vi "Frame.Dialog.vi"(6 "Signals":T1[](array[typedef]) {"Byte Order" items=["Little Endian", "Big Endian"]; "Data Type" items=["Signed", "Unsigned", "IEEE Float"]}, 7 "Show Name&ID":bool=TRUE, 8 "error in (no error)":errorcluster, 9 "ID":u16=1 caption="ID/Address" min=1 format="%.0x", 10 "Existing PIDs":string[](array[string]), 11 "Name":string) -> (0 "error out":errorcluster, 1 "ID out":u16=1 min=1 format="%.0x", 2 "Cancel PID?":bool, 3 "Name out":string, 4 "Signals out":T1[](array[typedef]) {"Byte Order" items=["Little Endian", "Big Endian"]; "Data Type" items=["Signed", "Unsigned", "IEEE Float"]})   [LabVIEW 2015, in "Diagnostics Addon System Explorer.lvlib"]
uses:
  Diagnostics Addon System Explorer.lvlib
  Shared/Types/Signal.ctl
  <vilib>/NI/AMC/Create Single Message.vi
  <vilib>/NI/AMC/Update Message Routing Info.vi
  <vilib>/NI/AMC/Read Termination Message.vi
  <vilib>/NI/AMC/Send Message.vi
  <vilib>/NI/AMC/Globals.vi
  Shared/Diagnostics Addon Shared.lvlib
  <vilib>/NI/AMC/AMC.lvlib
panel:
  in  "Default":dbl format="%g"
  in  "Units":string
  in  "Endian":u8(ring) items=["Little", "Big"]
  in  "Datatype":u8(ring)=1 items=["Signed", "Unsigned", "Float"]
  in  "Remove":bool
  in  "Add":bool
  in  "Cancel PID":bool
  in  "Apply":bool
  in  "Cancel":bool
  in  "OK":bool
  in  "Maximum":dbl=255.0 format="%g"
  in  "Minimum":dbl format="%g"
  in  "Offset":dbl format="%g"
  in  "Factor":dbl=1.0 format="%g"
  in  "Length":u32=8
  in  "Start Bit":u32
  in  "Signal Name":string
  in  "Signals":i32(listbox)
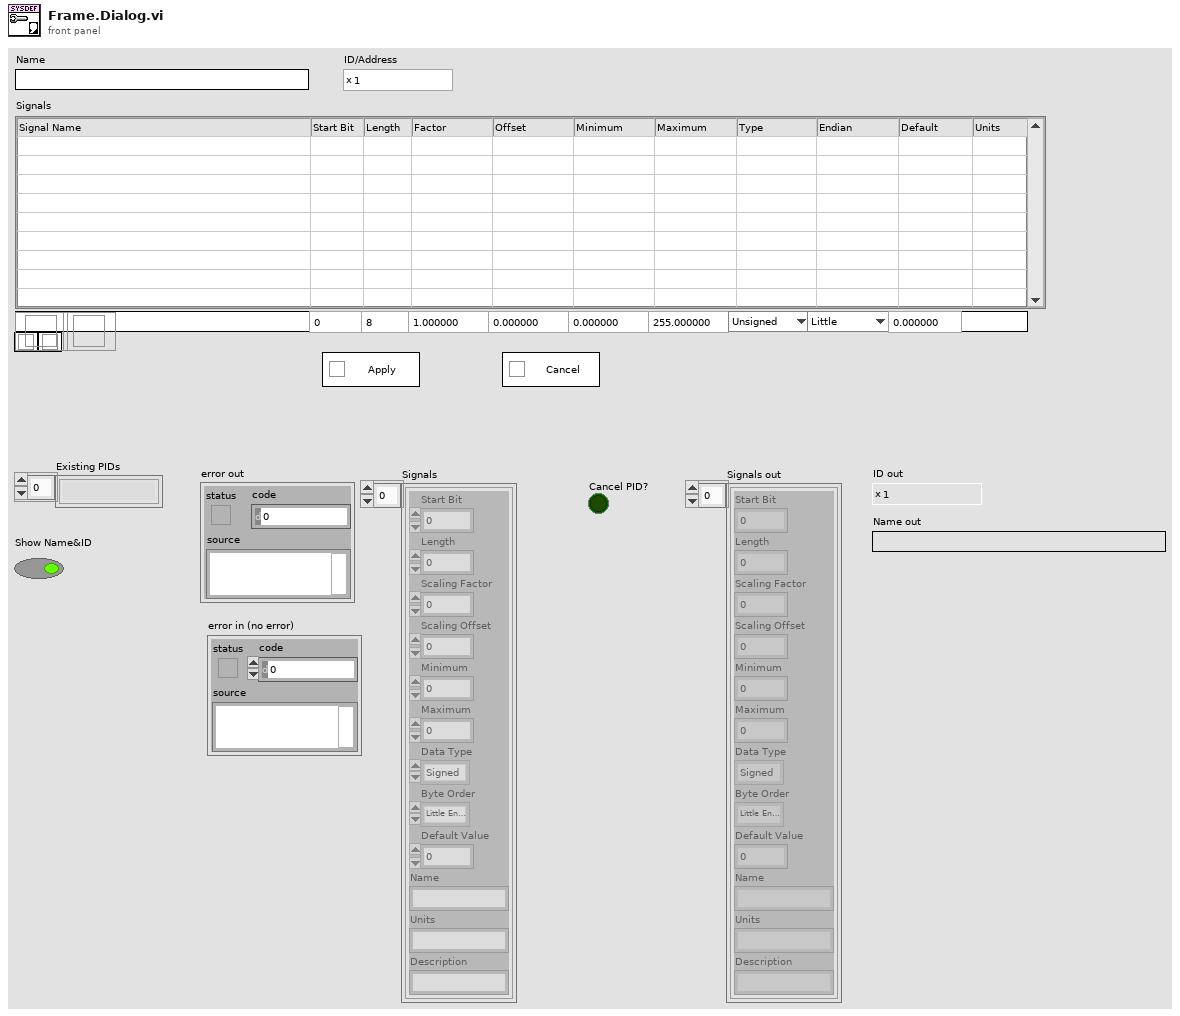
[diagram p1: front panel]
types:
  T1 = typedef "Diagnostics Addon Shared.lvlib/Signal.ctl" = cluster{"Start Bit":u32, "Length":u32, "Scaling Factor":dbl, "Scaling Offset":dbl, "Minimum":dbl, "Maximum":dbl, "Data Type":u32, "Byte Order":u32, "Default Value":dbl, "Name":string, "Units":string, "Description":string}
  T2 = cluster{"NewControlRefs":refnum<vi>[], "Add":refnum<vi>, "Listbox":refnum<vi>, "Remove":refnum<vi>, "Apply":refnum<vi>, "Cancel PID":refnum<vi>}
  T3 = typedef "AMC.lvlib/Message Queue.ctl" = refnum<queue>
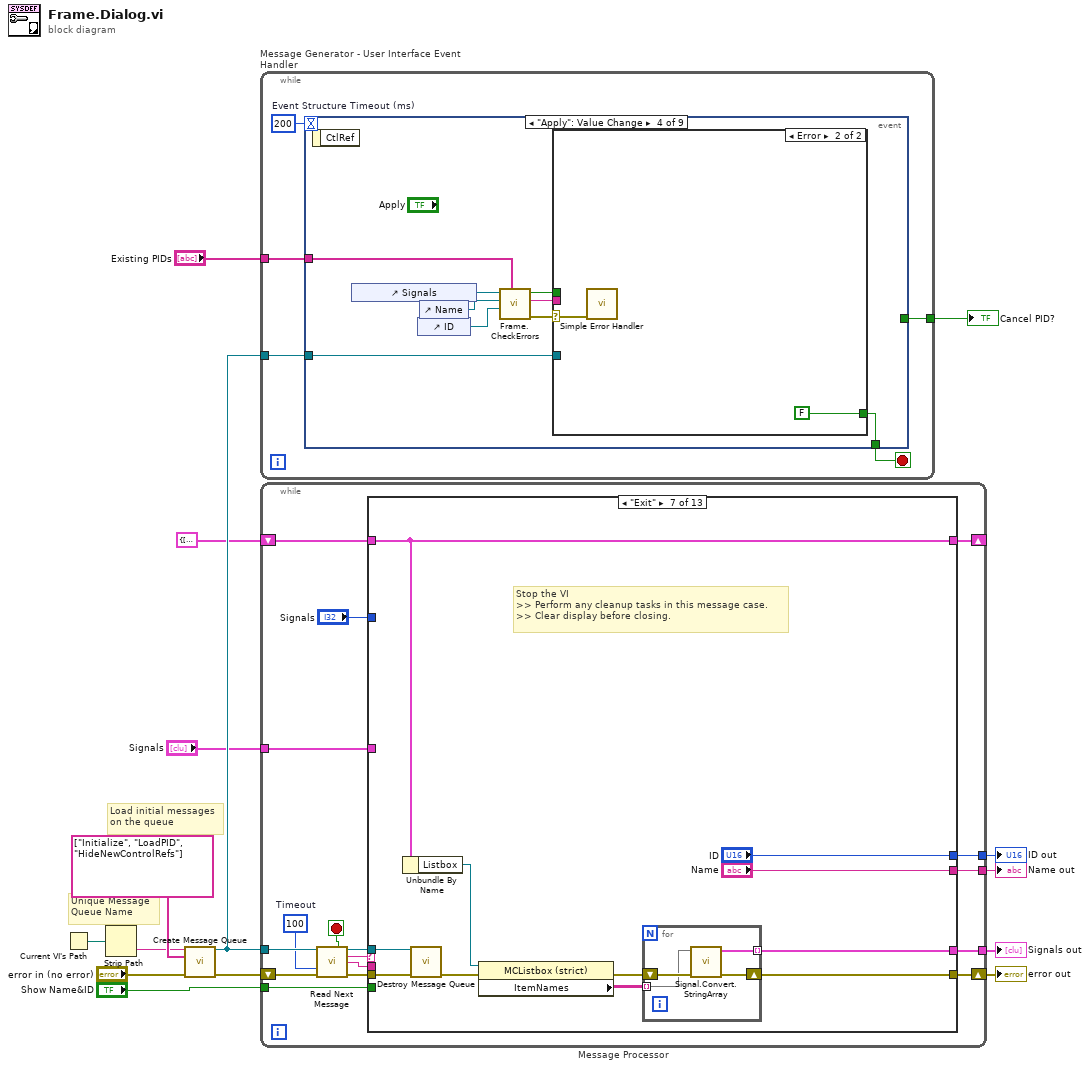
[diagram p0: block diagram]
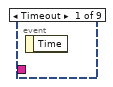
[diagram p2: hidden frame]
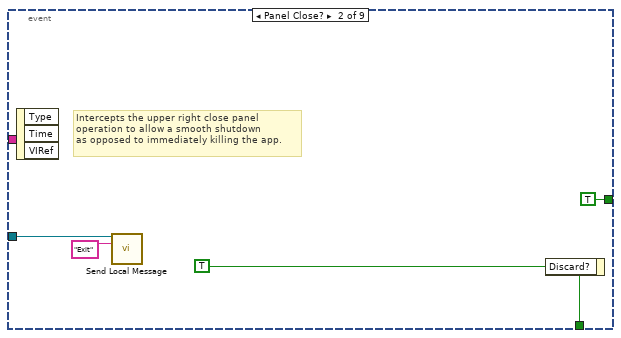
[diagram p3: hidden frame]
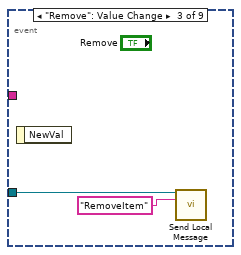
[diagram p4: hidden frame]
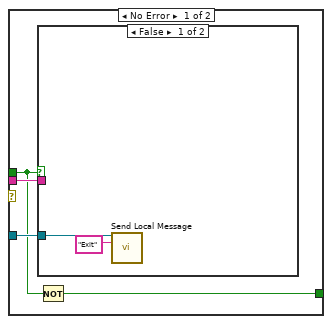
[diagram p5: hidden frame]
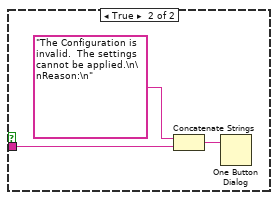
[diagram p6: hidden frame]
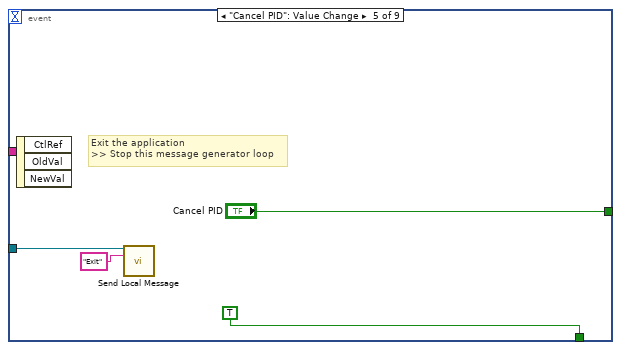
[diagram p7: hidden frame]
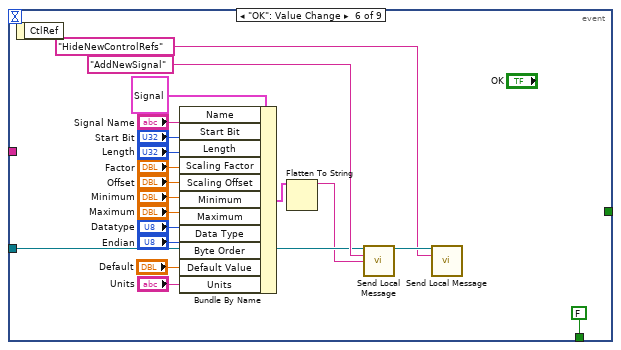
[diagram p8: hidden frame]
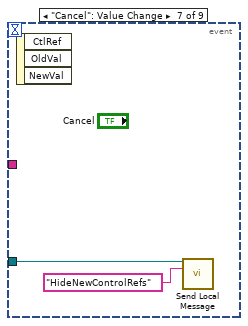
[diagram p9: hidden frame]
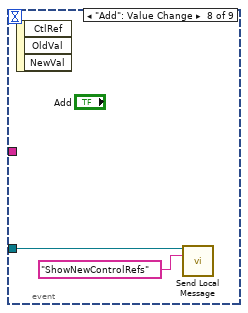
[diagram p10: hidden frame]
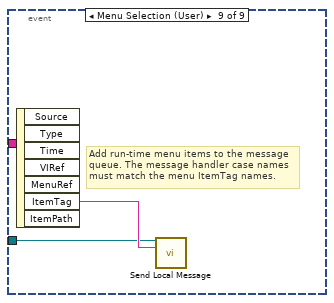
[diagram p11: hidden frame]
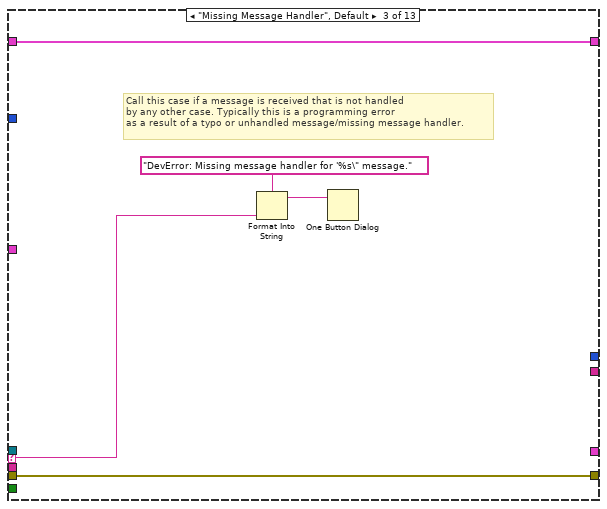
[diagram p14: hidden frame]
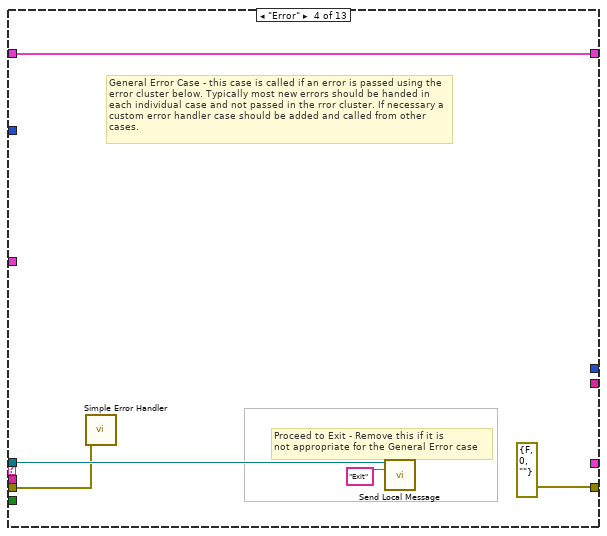
[diagram p15: hidden frame]
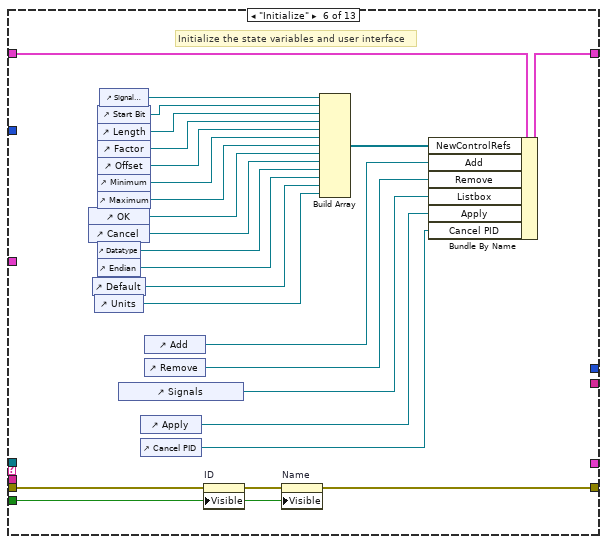
[diagram p17: hidden frame]
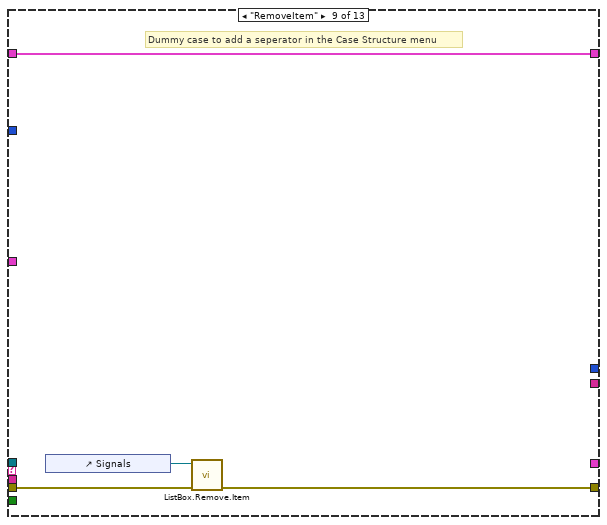
[diagram p19: hidden frame]
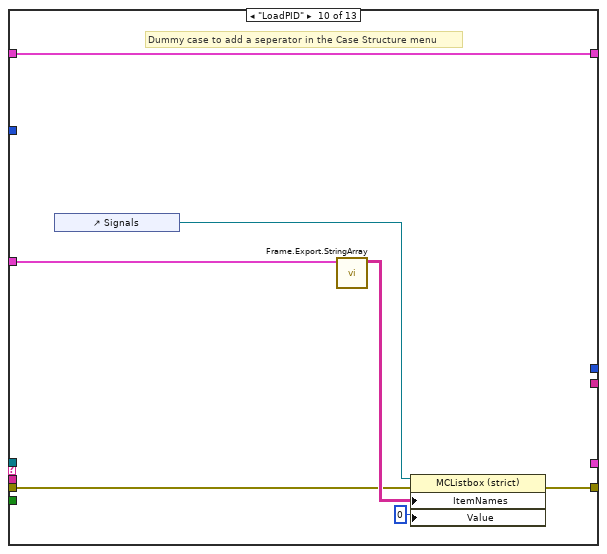
[diagram p20: hidden frame]
diagram:
  # "Unique Message\nQueue Name"
  # "Load initial messages\non the queue"
  n1 = Current VI's Path() -> (path=w11:path)
  n2 = Strip Path(path=w11) -> (name=w14:string)  [unwired: 1 out]
  n3 = call <vilib>:"Create Message Queue.vi"("message queue name"=w14, "initial message names"=string[] ["Initialize", "LoadPID", "HideNewControlRefs"], "error in"="error in (no error)") -> ("message queue out"=w13:T3, "error out"=w12:errorcluster)  [unwired: 11 in]
  n4 = while "Message Generator - User Interface Event Handler" {
    tunnel: w13 -> [w18]
    tunnel: [w17] -> w9
    tunnel: "Existing PIDs" -> [w16]
    stop <- w19 stop-if-true
    w20 = 200  # Event Structure Timeout (ms)
    n5 = event shown="[3] \"Apply\": Value Change" {
      selector: _ -> [_ _ _ _ _ _ _ _ _]
      dyn-events: _ -> [_ _ _ _ _ _ _ _ _]
      timeout: w20 -> [_ _ _ _ _ _ _ _ _]
      tunnel: [_ w24 _ w27 TRUE ("Discard?") FALSE ("Discard?") _ _ _] -> w19
      tunnel: w18 -> [_ w22 w25 w33 w48 w67 w70 w72 w74]
      tunnel: [_ TRUE ("Cancel PID") _ _ "Cancel PID" _ _ _ _] -> w17
      tunnel: w16 -> [_ _ _ w30 _ _ _ _ _]
      event Timeout {
        n6 = event-data() -> ()  [unwired: 2 out]
      }
      event Panel Close? {
        w24 = TRUE ("Discard?")
        # "Intercepts the upper right close panel\noperation to allow a smooth shutdown\nas opposed to immediately killing the app."
        n7 = event-data() -> ()  [unwired: 4 out]
        n8 = call <vilib>:"Send Local Message.vi"("message queue in"=w22, "message name"="Exit") -> ()  [unwired: 11 in, 3 out]
        n9 = event-data("Discard?"=w24) -> ()  [unwired: 1 in, 1 out]
      }
      event "Remove": Value Change {
        n10 = event-data() -> ()  [unwired: 2 out]
        n11 = call <vilib>:"Send Local Message.vi"("message queue in"=w25, "message name"="RemoveItem") -> ()  [unwired: 11 in, 3 out]
      }
      event "Apply": Value Change {
        n12 = event-data() -> ()  [unwired: 2 out]
        n13 = control-ref of="Signals"() -> (w35:refnum<vi>)
        n14 = control-ref of="ID"() -> (w31:refnum<vi>)
        n15 = control-ref of="Name"() -> (w32:refnum<vi>)
        n16 = call "Frame.CheckErrors.vi"("Existing PIDs"=w30, "ID"=w31, "Name"=w32, "Listbox"=w35) -> ("error out"=w28:errorcluster, "Error Type"=w29:string, "Error?"=w34:bool)  [unwired: 5 in]
        n17 = case shown="Error" w28 {
          selector: w28 -> [_ w46]
          tunnel: w34 -> [w37 _]
          tunnel: w33 -> [w39 _]
          tunnel: w29 -> [w38 _]
          tunnel: [w36 FALSE] -> w27
          frame No Error {
            n18 = case shown="False" w37 {
              tunnel: w39 -> [w41 _]
              tunnel: w38 -> [_ w44]
              frame False {
                n19 = call <vilib>:"Send Local Message.vi"("message queue in"=w41, "message name"="Exit" ("Message Name")) -> ()  [unwired: 11 in, 3 out]
              }
              frame True {
                n20 = Concatenate Strings("The Configuration is invalid.  The settings cannot be applied.\n\nReason:\n" ("message"), w44) -> (w42:string)
                n21 = One Button Dialog(message=w42) -> ()  [unwired: 1 in, 1 out]
              }
            }
            n22 = Not(x=w37) -> (.not. x?=w36:bool)
          }
          frame Error {
            n23 = call <vilib>:"Simple Error Handler.vi"("error in (no error)"=w46) -> ()  [unwired: 4 in, 5 out]
          }
        }
      }
      event "Cancel PID": Value Change {
        # "Exit the application\n>> Stop this message generator loop"
        n24 = event-data() -> ()  [unwired: 4 out]
        n25 = call <vilib>:"Send Local Message.vi"("message queue in"=w48, "message name"="Exit") -> ()  [unwired: 11 in, 3 out]
      }
      event "OK": Value Change {
        n26 = event-data() -> ()  [unwired: 2 out]
        n27 = Bundle By Name(cluster=T1 {"Start Bit"=0, "Length"=0, "Scaling Factor"=0.0, "Scaling Offset"=0.0, "Minimum"=0.0, "Maximum"=0.0, "Data Type"=0, "Byte Order"=0, "Default Value"=0.0, "Name"="", "Units"="", "Description"=""} ("Signal Parameters"), "Name"="Signal Name", "Start Bit"="Start Bit", "Length"="Length", "Scaling Factor"="Factor", "Scaling Offset"="Offset", "Minimum"="Minimum", "Maximum"="Maximum", "Data Type"="Datatype", "Byte Order"="Endian", "Default Value"="Default", "Units"="Units") -> (w58:T1)
        n28 = Flatten To String(anything=w58) -> (data string=w57:string)  [unwired: 3 in, 2 out]
        n29 = call <vilib>:"Send Local Message.vi"("message queue in"=w67, "message name"="AddNewSignal", "message value"=w57) -> ("message queue out"=w56:T3)  [unwired: 10 in, 2 out]
        n30 = call <vilib>:"Send Local Message.vi"("message queue in"=w56, "message name"="HideNewControlRefs" ("Message Name")) -> ()  [unwired: 11 in, 3 out]
      }
      event "Cancel": Value Change {
        n31 = event-data() -> ()  [unwired: 4 out]
        n32 = call <vilib>:"Send Local Message.vi"("message queue in"=w70, "message name"="HideNewControlRefs" ("Message Name")) -> ()  [unwired: 11 in, 3 out]
      }
      event "Add": Value Change {
        n33 = event-data() -> ()  [unwired: 4 out]
        n34 = call <vilib>:"Send Local Message.vi"("message queue in"=w72, "message name"="ShowNewControlRefs" ("Message Name")) -> ()  [unwired: 11 in, 3 out]
      }
      event Menu Selection (User) {
        # "Add run-time menu items to the message\nqueue. The message handler case names must match the menu ItemTag names."
        n35 = event-data() -> ("ItemTag"=w75:string)  [unwired: 7 out]
        n36 = call <vilib>:"Send Local Message.vi"("message queue in"=w74, "message name"=w75) -> ()  [unwired: 11 in, 3 out]
      }
    }
  }
  "Cancel PID?" <- w9
  n37 = while "Message Processor" {
    shift-left: w12 -> [w86]
    shift-right: [w90] -> w7
    tunnel: w13 -> [w87]
    shift-left: T2 {"NewControlRefs"=[], "Add"=refnum, "Listbox"=refnum, "Remove"=refnum, "Apply"=refnum, "Cancel PID"=refnum} ("State Variables") -> [w92]
    shift-right: [w91] -> _
    tunnel: "Signals" -> [w80]
    tunnel: [w79] -> w4
    tunnel: [w78] -> w3
    tunnel: [w77] -> w2
    tunnel: "Show Name&ID" -> [w76]
    stop <- w89 stop-if-true
    w84 = 100  # Timeout
    n38 = call <vilib>:"Read Next Message.vi"("message queue in"=w87, "timeout (1 ms)"=w84, "error in"=w86) -> ("exit process?"=w89:bool, "message queue out"=w88:T3, "message name"=w83:string, "message value"=w82:string, "error out"=w85:errorcluster)  [unwired: 5 in, 3 out]
    n39 = case shown="\"Exit\"" w83 {
      selector: w83 -> [_ _ w99 _ _ _ _ _ _ _ _ _ _]
      tunnel: [w94 w96 w101 w106 w108 w122 w142 w150 w154 w161 w167 w184 w198] -> w91
      tunnel: w92 -> [w94 w96 w101 w106 w108 w123 w142 w150 w154 w161 w167 w184 w198]
      tunnel: w88 -> [_ _ _ w104 _ _ w143 _ _ _ _ _ _]
      tunnel: w85 -> [w93 w95 w100 w102 w107 w113 w144 w149 w152 w155 w170 w183 w197]
      tunnel: [w93 w95 w100 errorcluster {"status"=FALSE, "code"=0, "source"=""} ("error out") w107 w112 w137 w149 w151 w158 w164 w173 w188] -> w90
      tunnel: w82 -> [_ _ _ _ _ _ _ _ _ _ w169 _ _]
      tunnel: "Signals" -> [_ _ _ _ _ _ _ _ _ _ _ _ _]
      tunnel: w80 -> [_ _ _ _ _ _ _ _ _ w156 _ _ _]
      tunnel: [_ _ _ _ _ _ w136 _ _ _ _ _ _] -> w79
      tunnel: [_ _ _ _ _ _ "Name" _ _ _ _ _ _] -> w78
      tunnel: [_ _ _ _ _ _ "ID" _ _ _ _ _ _] -> w77
      tunnel: w76 -> [_ _ _ _ _ w111 _ _ _ _ _ _ _]
      frame "---------- Framework Operations ----------" {
        # "Dummy case to add a seperator in the Case Structure menu"
      }
      frame "", "Idle" {
        # "Idle Case - this case is called after a Timeout on the Get Next Message from Queue VI, if no new messages are present on the queue. This case can be used for housekeeping tasks such as updating the UI."
      }
      frame "Missing Message Handler", Default {
        # "Call this case if a message is received that is not handled \nby any other case. Typically this is a programming error\nas a result of a typo or unhandled message/missing message handler."
        n40 = Format Into String(format string="DevError: Missing message handler for '%s\" message." ("message"), w99) -> (resulting string=w97:string)  [unwired: 2 in, 1 out]
        n41 = One Button Dialog(message=w97) -> ()  [unwired: 2 out]
      }
      frame "Error" {
        # "Proceed to Exit - Remove this if it is\nnot appropriate for the General Error case"
        # "General Error Case - this case is called if an error is passed using the error cluster below. Typically most new errors should be handed in each individual case and not passed in the rror cluster. If necessary a custom error handler case should be added and called from other cases."
        n42 = call <vilib>:"Simple Error Handler.vi"("error in (no error)"=w102) -> ()  [unwired: 1 in, 8 out]
        n43 = call <vilib>:"Send Local Message.vi"("message queue in"=w104, "message name"="Exit") -> ()  [unwired: 11 in, 3 out]
      }
      frame "---------- Generic Operations ----------" {
        # "Dummy case to add a seperator in the Case Structure menu"
      }
      frame "Initialize" {
        # "Initialize the state variables and user interface"
        n44 = control-ref of="OK"() -> (w132:refnum<vi>)
        n45 = control-ref of="Cancel"() -> (w133:refnum<vi>)
        n46 = control-ref of="Default"() -> (w110:refnum<vi>)
        n47 = control-ref of="Units"() -> (w109:refnum<vi>)
        n48 = control-ref of="Start Bit"() -> (w126:refnum<vi>)
        n49 = control-ref of="Length"() -> (w127:refnum<vi>)
        n50 = control-ref of="Factor"() -> (w128:refnum<vi>)
        n51 = control-ref of="Offset"() -> (w129:refnum<vi>)
        n52 = control-ref of="Minimum"() -> (w130:refnum<vi>)
        n53 = control-ref of="Maximum"() -> (w131:refnum<vi>)
        n54 = control-ref of="Datatype"() -> (w118:refnum<vi>)
        n55 = control-ref of="Endian"() -> (w117:refnum<vi>)
        n56 = control-ref of="Signal Name"() -> (w125:refnum<vi>)
        n57 = control-ref of="Signals"() -> (w120:refnum<vi>)
        n58 = control-ref of="Apply"() -> (w116:refnum<vi>)
        n59 = control-ref of="Cancel PID"() -> (w115:refnum<vi>)
        n60 = control-ref of="Add"() -> (w121:refnum<vi>)
        n61 = control-ref of="Remove"() -> (w119:refnum<vi>)
        n62 = property on="ID" class="DigNum (strict)"(error in=w113, "Visible"=w111) -> (error out=w114:errorcluster)  [unwired: 1 in, 1 out]
        n63 = property on="Name" class="Str"(error in=w114, "Visible"=w111) -> (error out=w112:errorcluster)  [unwired: 1 in, 1 out]
        n64 = Build Array(w125, w126, w127, w128, w129, w130, w131, w132, w133, w118, w117, w110, w109) -> (w124:refnum<vi>[])
        n65 = Bundle By Name(cluster=w123, "NewControlRefs"=w124, "Add"=w121, "Remove"=w119, "Listbox"=w120, "Apply"=w116, "Cancel PID"=w115) -> (w122:T2)
      }
      frame "Exit" {
        # "Stop the VI\n>> Perform any cleanup tasks in this message case.\n>> Clear display before closing."
        n66 = Unbundle By Name(w142) -> ("Listbox"=w141:refnum<vi>)
        n67 = call <vilib>:"Destroy Message Queue.vi"("message queue in"=w143, "error in"=w144) -> ("error out"=w140:errorcluster)  [unwired: 11 in, 2 out]
        n68 = property class="MCListbox (strict)"(reference=w141, error in=w140) -> (error out=w138:errorcluster, "ItemNames"=w139:string[][])  [unwired: 1 out]
        n69 = for {
          shift-right: [w147] -> w137
          shift-left: w138 -> [w148]
          tunnel: w139 -> [w146] mode=indexing
          tunnel: [w145] -> w136 mode=indexing
          n70 = call "Signal.Convert.StringArray.vi"("error in (no error)"=w148, "Signal Parameters"=w146) -> ("error out"=w147:errorcluster, "Signal Parameters"=w145:T1)  [unwired: 8 in]
        }
      }
      frame "---------- Application Operations ----------" {
        # "Dummy case to add a seperator in the Case Structure menu"
      }
      frame "RemoveItem" {
        # "Dummy case to add a seperator in the Case Structure menu"
        n71 = control-ref of="Signals"() -> (w153:refnum<vi>)
        n72 = call "ListBox.Remove.Item.vi"("error in (no error)"=w152, "MulticolumnListbox in"=w153) -> ("error out"=w151:errorcluster)  [unwired: 9 in]
      }
      frame "LoadPID" {
        # "Dummy case to add a seperator in the Case Structure menu"
        n73 = control-ref of="Signals"() -> (w160:refnum<vi>)
        n74 = call "Frame.Export.StringArray.vi"("Frame Parameters"=w156) -> ("Frame Parameters"=w157:string[][])  [unwired: 9 in, 1 out]
        n75 = property class="MCListbox (strict)"(reference=w160, error in=w155, "ItemNames"=w157, "Value"=0) -> (error out=w158:errorcluster)  [unwired: 1 out]
      }
      frame "AddNewSignal" {
        # "Dummy case to add a seperator in the Case Structure menu"
        n76 = Unflatten From String(type=T1 {"Start Bit"=0, "Length"=0, "Scaling Factor"=0.0, "Scaling Offset"=0.0, "Minimum"=0.0, "Maximum"=0.0, "Data Type"=0, "Byte Order"=0, "Default Value"=0.0, "Name"="", "Units"="", "Description"=""} ("Signal Parameters"), binary string=w169, error in (no error)=w170) -> (value=w163:T1, error out=w165:errorcluster)  [unwired: 2 in, 1 out]
        n77 = Unbundle By Name(w167) -> ("Listbox"=w166:refnum<vi>)
        n78 = call "Signal.Export.StringArray.vi"("Signal Parameters"=w163) -> ("Array"=w162:string[])  [unwired: 10 in]
        n79 = call "Listbox.Add.Item.vi"("error in (no error)"=w165, "Item"=w162, "MulticolumnListbox in"=w166) -> ("error out"=w164:errorcluster)  [unwired: 8 in]
      }
      frame "HideNewControlRefs" {
        w175 = TRUE ("Visible")
        # "Dummy case to add a seperator in the Case Structure menu"
        n80 = Unbundle By Name(w184) -> ("Cancel PID"=w171:refnum<vi>, "Apply"=w172:refnum<vi>, "Remove"=w177:refnum<vi>, "Add"=w179:refnum<vi>, "NewControlRefs"=w182:refnum<vi>[])
        n81 = call "Controls.Set.Visible.vi"("error in"=w183, "Visible?"=FALSE, "Control Refs"=w182) -> ("error out"=w180:errorcluster)  [unwired: 8 in]
        n82 = property class="Bool"(reference=w179, error in=w180, "Visible"=w175) -> (error out=w178:errorcluster)  [unwired: 1 out]
        n83 = property class="Bool"(reference=w177, error in=w178, "Visible"=w175) -> (error out=w174:errorcluster)  [unwired: 1 out]
        n84 = property class="Bool"(reference=w172, error in=w174, "Visible"=w175) -> (error out=w176:errorcluster)  [unwired: 1 out]
        n85 = property class="Bool"(reference=w171, error in=w176, "Visible"=w175) -> (error out=w173:errorcluster)  [unwired: 1 out]
      }
      frame "ShowNewControlRefs" {
        w187 = FALSE ("Visible")
        # "Dummy case to add a seperator in the Case Structure menu"
        n86 = Unbundle By Name(w198) -> ("Apply"=w186:refnum<vi>, "Cancel PID"=w185:refnum<vi>, "Remove"=w191:refnum<vi>, "Add"=w193:refnum<vi>, "NewControlRefs"=w196:refnum<vi>[])
        n87 = call "Controls.Set.Visible.vi"("error in"=w197, "Visible?"=TRUE, "Control Refs"=w196) -> ("error out"=w194:errorcluster)  [unwired: 8 in]
        n88 = property class="Bool"(reference=w193, error in=w194, "Visible"=w187) -> (error out=w192:errorcluster)  [unwired: 1 out]
        n89 = property class="Bool"(reference=w191, error in=w192, "Visible"=w187) -> (error out=w189:errorcluster)  [unwired: 1 out]
        n90 = property class="Bool"(reference=w185, error in=w189, "Visible"=w187) -> (error out=w190:errorcluster)  [unwired: 1 out]
        n91 = property class="Bool"(reference=w186, error in=w190, "Visible"=w187) -> (error out=w188:errorcluster)  [unwired: 1 out]
      }
    }
  }
  "error out" <- w7
  "Signals out" <- w4
  "ID out" <- w2
  "Name out" <- w3
